vi "ACT_Loop.vi"() -> ()   [LabVIEW 2020, in "Wrist_ACT.lvlib"]
uses:
  Wrist_ACT.lvlib
  Cluster_CMD_ACT_Data.ctl
  Shared Code/TypeDefs/ENUM_Wrist_CMD_Mode Select.ctl
  Shared Code/TypeDefs/Cluster_Wrist_Config HW Values.ctl
  Shared Code/TypeDefs/Cluser_CAN Data.ctl
  Shared Code/TypeDefs/Cluster_Config Motor Output.ctl
  <vilib>/Rock Robotics/WPI/ThirdParty/Phoenix-LabVIEW/Motor Controller/Controls/CTRE_Phoenix_MotorControl_TalonFXInvertType.ctl
  <vilib>/Rock Robotics/WPI/ThirdParty/Phoenix-LabVIEW/Motor Controller/Controls/CTRE_Phoenix_MotorControl_NeutralMode.ctl
  Shared Code/TypeDefs/Cluster_FWD  REV Values.ctl
  Shared Code/TypeDefs/Cluster_PID Config.ctl
  Shared Code/TypeDefs/Cluster_PID Gains.ctl
  Shared Code/TypeDefs/Cluster_High-Low.ctl
  Shared Code/TypeDefs/Cluster_Motion Magic Parameters.ctl
  Shared Code/TypeDefs/Cluser_Limit Travel Config.ctl
  Shared Code/TypeDefs/Cluser_Hard Limits.ctl
  <vilib>/Rock Robotics/WPI/ThirdParty/Phoenix-LabVIEW/Motor Controller/Controls/CTRE_Phoenix_MotorControl_LimitSwitchNormal.ctl
  Shared Code/TypeDefs/Cluser_Config_Soft Limits.ctl
  Shared Code/TypeDefs/Cluser_Enable-Value I32.ctl
  Shared Code/TypeDefs/Cluster_Config_Cancoder Data.ctl
  Shared Code/TypeDefs/Cluser_Config_Current Limits.ctl
  Shared Code/TypeDefs/Cluster_Wrist HW Outputs.ctl
  Shared Code/TypeDefs/Cluster_FX Sensor Values.ctl
  Shared Code/TypeDefs/Cluster_FX CloseLoop Values.ctl
  Shared Code/TypeDefs/Cluster_FX Limit Switchs.ctl
  Shared Code/TypeDefs/Cluster_FX Current Values.ctl
  Shared Code/TypeDefs/Cluster_FX Integrated Sensor Values.ctl
  Shared Code/TypeDefs/Cluster_Wrist_SW Output Data.ctl
  Shared Code/TypeDefs/Cluster_Wrist_Config SW Values.ctl
  ENUM_ACT_State.ctl
  <vilib>/Rock Robotics/WPI/MotorControl/WPI_MotorControlDeviceRef.ctl
  <vilib>/Rock Robotics/WPI/MotorControl/WPI_MotorControlType.ctl
  <vilib>/Rock Robotics/SystemInterfaces/DIO/FPGA_DIOPWMChannel.ctl
  <vilib>/Rock Robotics/WPI/PWM/WPI_PWMDeadband.ctl
  <vilib>/Rock Robotics/SystemInterfaces/DIO/FPGA_DIOChannel.ctl
  <vilib>/Rock Robotics/WPI/ThirdParty/Phoenix-LabVIEW/Motor Controller/Controls/CTRE_Phoenix_MotorControl_ControlMode.ctl
  <vilib>/Rock Robotics/WPI/ThirdParty/Phoenix-LabVIEW/CANCoder/Controls/CTRE_Phoenix_CANcoder_DeviceRef.ctl
  ENUM_ACT_Action.ctl
  b65afb20-a57c-4a75-aa10-15f74f40a4cd.vi
  e7fa0f6b-fe57-4250-9995-b404d65a8362.vi
  4f1f8321-3dc8-4b28-8619-20673fc77ec2.vi
  6201c2b1-dcd8-4430-86f1-9b4ee56c7753.vi
  b5508d6c-c1cc-4273-80c5-2077d34e1483.vi
  36677ea0-a1a5-47a3-bc56-4475cb7c281e.vi
  5f725c2a-0ce1-4524-8967-e83b15fdce90.vi
  573e44c0-11f4-4bd9-ad56-904ec25dba75.vi
  e7494af9-f670-4352-9dfa-ae6ce50709ea.vi
  36677ea0-a1a5-47a3-bc56-4475cb7c281e.vi/f38ca901-adc1-4ad8-996e-31aeb746ae36.vi
  36677ea0-a1a5-47a3-bc56-4475cb7c281e.vi/958b2683-dd4b-41b7-8ed1-41c95f63cef0.vi
  5f725c2a-0ce1-4524-8967-e83b15fdce90.vi/f38ca901-adc1-4ad8-996e-31aeb746ae36.vi
  5f725c2a-0ce1-4524-8967-e83b15fdce90.vi/958b2683-dd4b-41b7-8ed1-41c95f63cef0.vi
  573e44c0-11f4-4bd9-ad56-904ec25dba75.vi/f38ca901-adc1-4ad8-996e-31aeb746ae36.vi
  573e44c0-11f4-4bd9-ad56-904ec25dba75.vi/958b2683-dd4b-41b7-8ed1-41c95f63cef0.vi
  e7494af9-f670-4352-9dfa-ae6ce50709ea.vi/f38ca901-adc1-4ad8-996e-31aeb746ae36.vi
  e7494af9-f670-4352-9dfa-ae6ce50709ea.vi/958b2683-dd4b-41b7-8ed1-41c95f63cef0.vi
  36677ea0-a1a5-47a3-bc56-4475cb7c281e.vi/f38ca901-adc1-4ad8-996e-31aeb746ae36.vi/1c6bd52c-bbca-4d4a-a290-93ea2703fded.vi
  36677ea0-a1a5-47a3-bc56-4475cb7c281e.vi/f38ca901-adc1-4ad8-996e-31aeb746ae36.vi/47c2b0d5-b5fa-444e-9535-611565d375db.vi
  5f725c2a-0ce1-4524-8967-e83b15fdce90.vi/f38ca901-adc1-4ad8-996e-31aeb746ae36.vi/1c6bd52c-bbca-4d4a-a290-93ea2703fded.vi
  5f725c2a-0ce1-4524-8967-e83b15fdce90.vi/f38ca901-adc1-4ad8-996e-31aeb746ae36.vi/47c2b0d5-b5fa-444e-9535-611565d375db.vi
  573e44c0-11f4-4bd9-ad56-904ec25dba75.vi/f38ca901-adc1-4ad8-996e-31aeb746ae36.vi/1c6bd52c-bbca-4d4a-a290-93ea2703fded.vi
  573e44c0-11f4-4bd9-ad56-904ec25dba75.vi/f38ca901-adc1-4ad8-996e-31aeb746ae36.vi/47c2b0d5-b5fa-444e-9535-611565d375db.vi
  e7494af9-f670-4352-9dfa-ae6ce50709ea.vi/f38ca901-adc1-4ad8-996e-31aeb746ae36.vi/1c6bd52c-bbca-4d4a-a290-93ea2703fded.vi
  e7494af9-f670-4352-9dfa-ae6ce50709ea.vi/f38ca901-adc1-4ad8-996e-31aeb746ae36.vi/47c2b0d5-b5fa-444e-9535-611565d375db.vi
  Utility/Global_STOP.vi
  Global_CMD_ACT_Data In.vi
  <vilib>/Utility/Data Type/Get Type Information.vi
  <vilib>/Utility/error.llb/Trim Whitespace.vi
  Shared Code/Utility/RWA/RWA/File/RWA_PC FIle Read String.vi
  Shared Code/Utility/RWA/RWA/Read Write Anything/RWA_File String.vi
  Shared Code/Utility/RWA/RWA/File/RWA_PC File Write String.vi
  <vilib>/Rock Robotics/WPI/ThirdParty/Phoenix-LabVIEW/CANCoder/Get/CTRE_Phoenix_CANcoder_GetSensorData.vi
  Global_ACT_Data Out.vi
  <vilib>/Comparison/Equal/Equal Functor/Equal Functor.lvclass
panel:
  in  "CMD Override":enum32{"None", "Velocity", "Position", "STOP"}(tab)
  in  "Velocity":dbl(slide) scale=-0.2..0.2
  in  "Target Counts":i32
  in  "Positon GO":bool
  out "Current Time":timestamp
  in  "SW Config":T1={"WristSW Ver"=0, "At Position Delay(S)"=0.2}
  out "SW Output":T2
  in  "Reset zero Offset on Limit Switch":bool
  out "Sensor Read time":dbl format="%.3g"
  out "HW Outputs":T3
  in  "Read Saved Config":bool
  in  "Update Config":bool
  in  "HW Config":T9 {"TravelLimits"."Soft"."REV"."Counts" format="%#.0f"; "TravelLimits"."Soft"."FWD"."Counts" format="%#.0f"; "Output"."Min"."REV" format="%.2f"; "Output"."Min"."FWD" format="%.2f"; "Output"."Max"."REV" format="%.2f"; "Output"."Max"."FWD" format="%.2f"; "CL"."Max I Accu"."Low" format="%#.8f"; "CL"."Max I Accu"."High" format="%#.8f"; "CL"."Gains"."F" format="%#.8f"; "CL"."Gains"."D" format="%#.8f"; "CL"."Gains"."I" format="%#.8f"; "CL"."Gains"."P" format="%#.8f"; "CL"."Error Allowed"."Low" format="%#.8f"; "CL"."Error Allowed"."High" format="%#.8f"; "CL"."I Zone"."Low" format="%#.8f"; "CL"."I Zone"."High" format="%#.8f"; "CL"."Max Out"."REV" format="%.2f"; "CL"."Max Out"."FWD" format="%.2f"}
  out "CMD":T26
  out "Cycle Time (S)":dbl format="%.3g"
  # "STOP"
  # "Tune Output\nto 1023 Max"
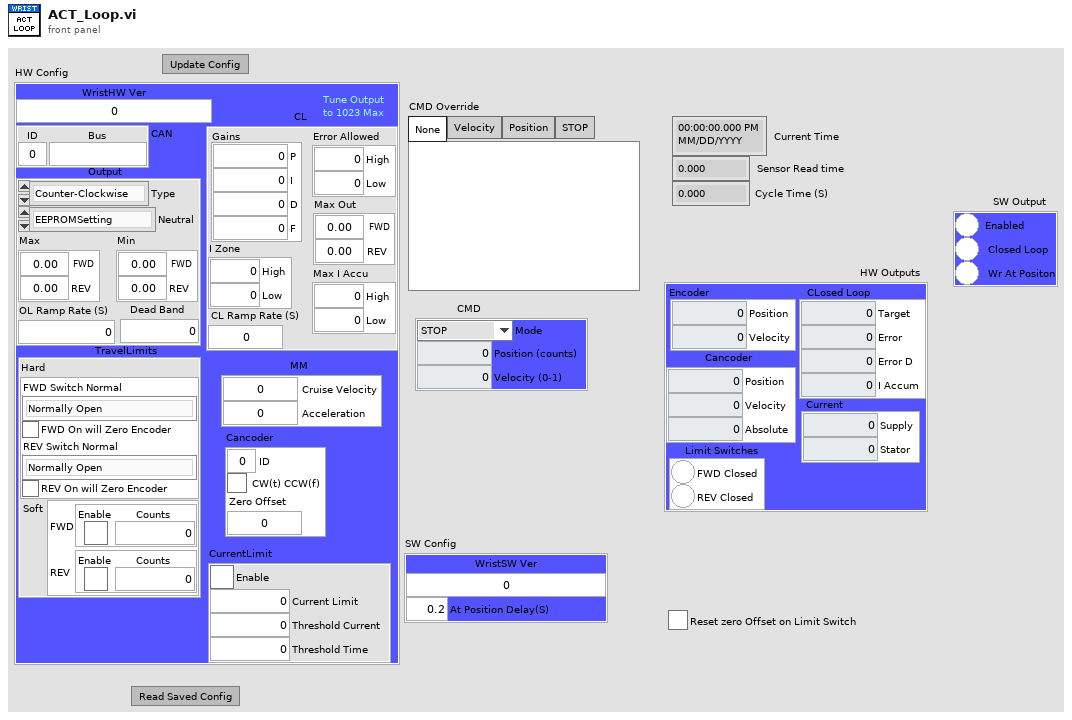
[diagram p1: front panel]
types:
  T1 = typedef "Cluster_Wrist_Config SW Values.ctl" = cluster{"WristSW Ver":u64, "At Position Delay(S)":dbl}
  T2 = typedef "Cluster_Wrist_SW Output Data.ctl" = cluster{"Enabled":bool, "Closed Loop":bool, "Wr At Positon":bool}
  T3 = typedef "Cluster_Wrist HW Outputs.ctl" = cluster{"Encoder":T4, "CLosed Loop":T5, "Limit Switches":T6, "Current":T7, "Cancoder":T8}
  T4 = typedef "Cluster_FX Sensor Values.ctl" = cluster{"Position":i32, "Velocity":i32}
  T5 = typedef "Cluster_FX CloseLoop Values.ctl" = cluster{"Target":dbl, "Error":i32, "Error D":dbl, "I Accum":dbl}
  T6 = typedef "Cluster_FX Limit Switchs.ctl" = cluster{"FWD Closed":bool, "REV Closed":bool}
  T7 = typedef "Cluster_FX Current Values.ctl" = cluster{"Supply":dbl, "Stator":dbl}
  T8 = typedef "Cluster_FX Integrated Sensor Values.ctl" = cluster{"Position":dbl, "Velocity":dbl, "Absolute":dbl}
  T9 = typedef "Cluster_Wrist_Config HW Values.ctl" = cluster{"WristHW Ver":u64, "CAN":T10, "Output":T11, "CL":T15, "MM":T18, "TravelLimits":T19, "Cancoder":T24, "CurrentLimit":T25}
  T10 = typedef "Cluser_CAN Data.ctl" = cluster{"ID":u8, "Bus":string}
  T11 = typedef "Cluster_Config Motor Output.ctl" = cluster{"Type":T12, "Neutral":T13, "Max":T14, "Min":T14, "OL Ramp Rate (S)":dbl, "Dead Band":dbl}
  T12 = typedef "CTRE_Phoenix_MotorControl_TalonFXInvertType.ctl" = enum16{"Counter-Clockwise", "Clockwise"}
  T13 = typedef "CTRE_Phoenix_MotorControl_NeutralMode.ctl" = enum8{"EEPROMSetting", "Override to Coast", "Override to Brake"}
  T14 = typedef "Cluster_FWD  REV Values.ctl" = cluster{"FWD":dbl, "REV":dbl}
  T15 = typedef "Cluster_PID Config.ctl" = cluster{"Gains":T16, "Error Allowed":T17, "I Zone":T17, "Max Out":T14, "Max I Accu":T17, "CL Ramp Rate (S)":dbl}
  T16 = typedef "Cluster_PID Gains.ctl" = cluster{"P":dbl, "I":dbl, "D":dbl, "F":dbl}
  T17 = typedef "Cluster_High-Low.ctl" = cluster{"High":dbl, "Low":dbl}
  T18 = typedef "Cluster_Motion Magic Parameters.ctl" = cluster{"Cruise Velocity":i32, "Acceleration":i32}
  T19 = typedef "Cluser_Limit Travel Config.ctl" = cluster{"Hard":T20, "Soft":T22}
  T20 = typedef "Cluser_Hard Limits.ctl" = cluster{"FWD Switch Normal":T21, "FWD On will Zero Encoder ":bool, "REV Switch Normal":T21, "REV On will Zero Encoder ":bool}
  T21 = typedef "CTRE_Phoenix_MotorControl_LimitSwitchNormal.ctl" = enum16{"Normally Open", "Normally Closed", "Disabled"}
  T22 = typedef "Cluser_Config_Soft Limits.ctl" = cluster{"FWD":T23, "REV":T23}
  T23 = typedef "Cluser_Enable-Value I32.ctl" = cluster{"Enable":bool, "Counts":i32}
  T24 = typedef "Cluster_Config_Cancoder Data.ctl" = cluster{"ID":u8, "CW(t) CCW(f)":bool, "Zero Offset":dbl}
  T25 = typedef "Cluser_Config_Current Limits.ctl" = cluster{"Enable":bool, "Current Limit":dbl, "Threshold Current":dbl, "Threshold Time":dbl}
  T26 = typedef "Wrist_ACT.lvlib/Cluster_CMD_ACT_Data.ctl" = cluster{"Mode":T27, "Position (counts)":i32, "Velocity (0-1)":dbl}
  T27 = typedef "ENUM_Wrist_CMD_Mode Select.ctl" = enum16{"STOP", "Position", "Speed"}
  T28 = typedef "CTRE_Phoenix_CANcoder_DeviceRef.ctl" = cluster{"DeviceStatus":errorcluster, "Device Number":u8, "Handle":u64, "UsageFrame":u32, "Library Path":path}
  T29 = typedef "CTRE_Phoenix_MotorControl_ControlMode.ctl" = u16
  T30 = typedef "WPI_MotorControlDeviceRef.ctl" = cluster{"DeviceStatus":errorcluster, "Type":T31, "PWM":cluster{"PWM Channel":T32, "DeadBand":T33}, "CAN":cluster{"Device Number":u8, "SetOutput VI Ref":variant, "GetOutput VI Ref":variant, "Enable VI Ref":variant, "Disable VI Ref":variant, "Data":variant}, "Invert":bool, "DIO PWM":cluster{"PWM \"Enable\" Channel":T32, "DIOChannel":T34, "PWM Rate":dbl}}
  T31 = typedef "WPI_MotorControlType.ctl" = enum16{"PWM", "CAN", "DIO PWM"}
  T32 = typedef "FPGA_DIOPWMChannel.ctl" = enum8{"PWM 0", "PWM 1", "PWM 2", "PWM 3", "PWM 4", "PWM 5", "PWM 6", "PWM 7", "PWM 8", "PWM 9", "PWM MXP 0", "PWM MXP 1", "PWM MXP 2", "PWM MXP 3", "PWM MXP 4", "PWM MXP 5", "PWM MXP 6", "PWM MXP 7", "PWM MXP 8", "PWM MXP 9", "Invalid"}
  T33 = typedef "WPI_PWMDeadband.ctl" = cluster{"Name":string, "maxPositivePwm":i32, "minPositivePwm":i32, "centerPwm":i32, "maxNegativePwm":i32, "minNegativePwm":i32, "angularRange":u16}
  T34 = typedef "FPGA_DIOChannel.ctl" = enum8{"DIO 0", "DIO 1", "DIO 2", "DIO 3", "DIO 4", "DIO 5", "DIO 6", "DIO 7", "DIO 8", "DIO 9", "DIO MXP 0", "DIO MXP 1", "DIO MXP 2", "DIO MXP 3", "DIO MXP 4", "DIO MXP 5", "DIO MXP 6", "DIO MXP 7", "DIO MXP 8", "DIO MXP 9", "DIO MXP 10", "DIO MXP 11", "DIO MXP 12", "DIO MXP 13", "DIO MXP 14", "DIO MXP 15", "SPI Port CS1", "SPI Port CS2", "SPI Port CS3", "SPI Port MISO", "SPI Port MOSI", "Invalid"}
  T35 = typedef "Wrist_ACT.lvlib/ENUM_ACT_State.ctl" = enum16{"Startup", "Configuring", "Stopping", "Moving Position", "Moving Velocity", "Shutdown"}
  T36 = cluster{"Falcon Ref":T30, "State":T35, "Previous State":T35, "Current Time":timestamp, "Previous Time":timestamp, "Start Time":timestamp, "Target Time (ms)":u32, "Cycle Time(S)":dbl, "ACT Input":T26, "ACT Output DBL":dbl, "Team Files Folder":path, "HW Config":T9, "Update Display":bool, "Max # Of Config Tries":i32, "CAN Timeout":u32, "FX Mode":T29, "FX Set Value":dbl, "HW Outputs":T3, "CANcoder Ref":T28, "SW Outputs":T2, "SW Config":T1}
  T37 = typedef "Wrist_ACT.lvlib/ENUM_ACT_Action.ctl" = enum16{"No Action", "Reset Time", "Reset All", "Config HW File Read", "Config HW File Save", "Config SW File Read", "Config SW File Save", "Config From FP", "Config HW Get", "Config HW Set", "Open HW Only", "Control FX Stop", "Control FX Positon", "Control FX Speed", "Config Cancoder Get Offset Value"}
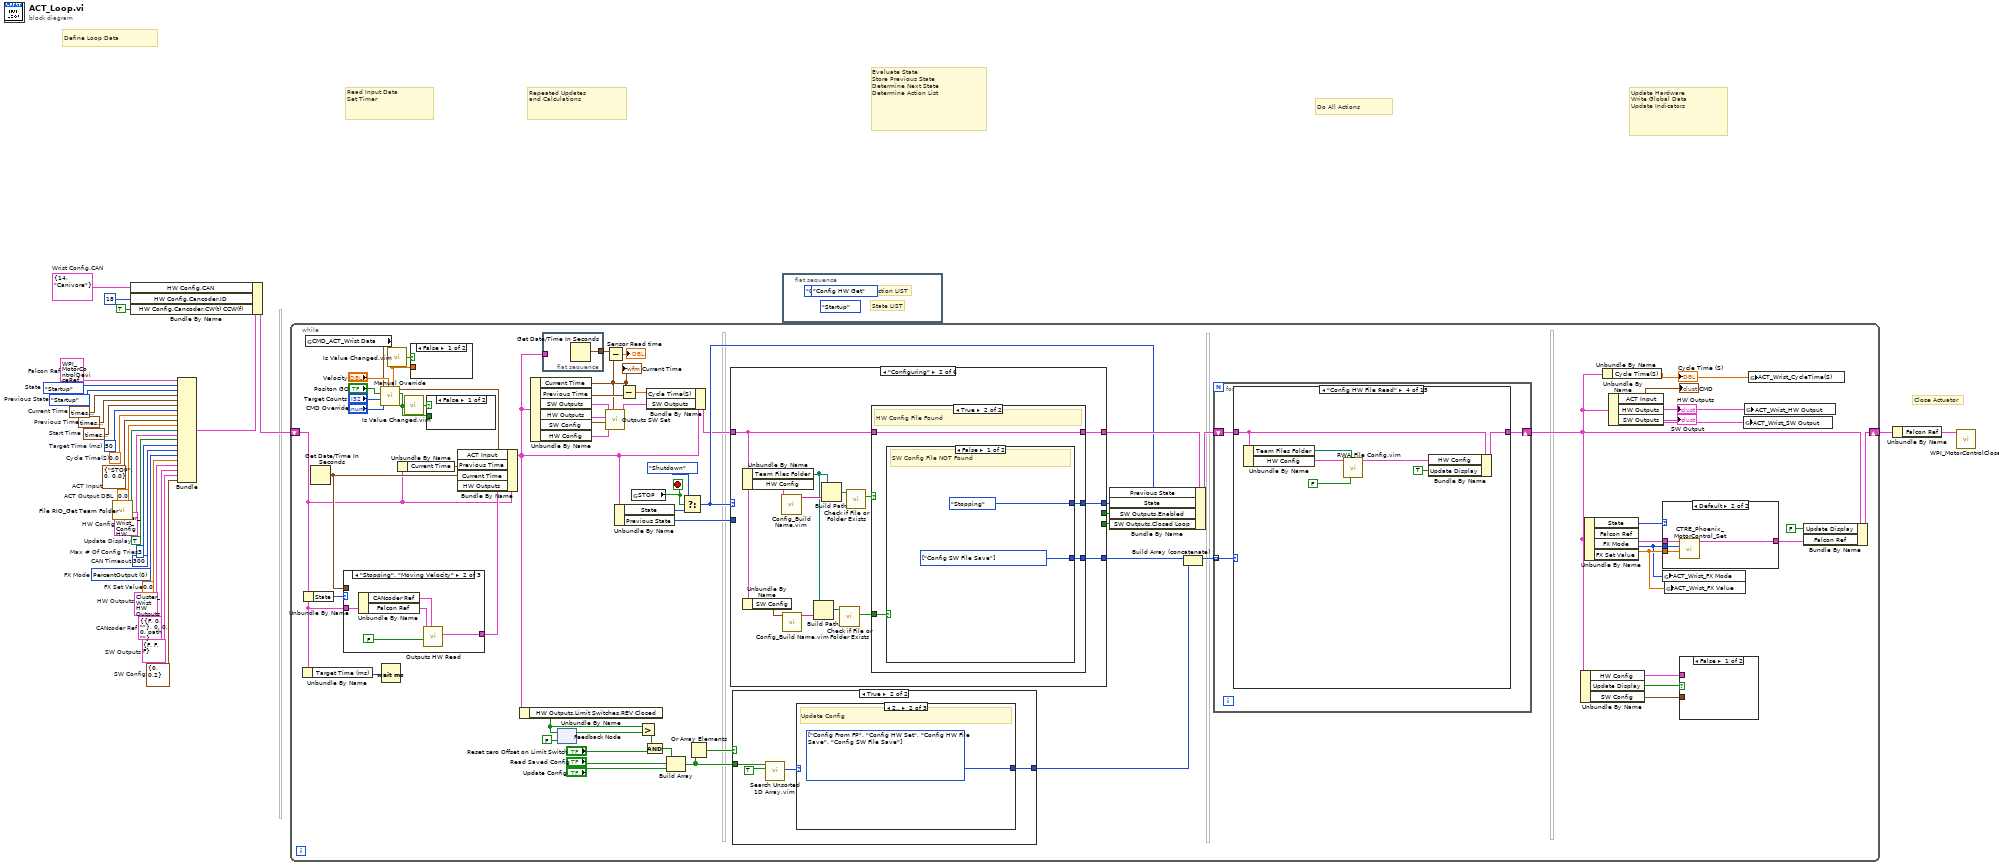
[diagram p0: block diagram]
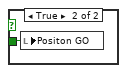
[diagram p2: hidden frame]
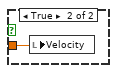
[diagram p3: hidden frame]
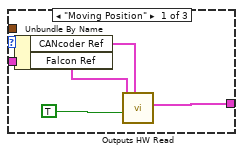
[diagram p4: hidden frame]
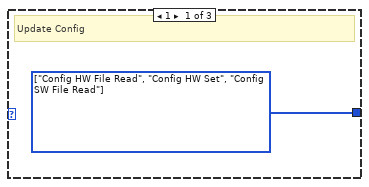
[diagram p7: hidden frame]
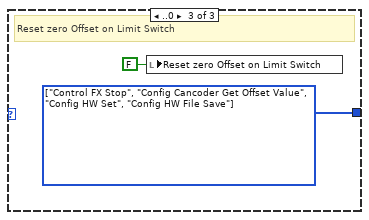
[diagram p8: hidden frame]
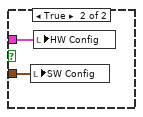
[diagram p10: hidden frame]
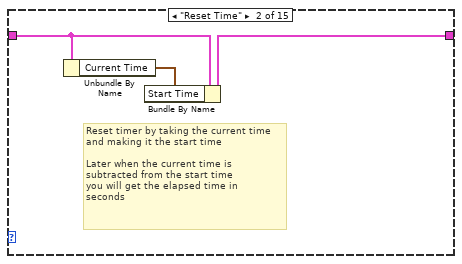
[diagram p12: hidden frame]
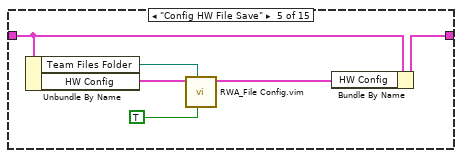
[diagram p14: hidden frame]
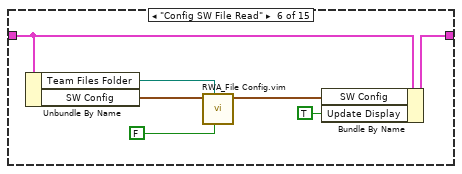
[diagram p15: hidden frame]
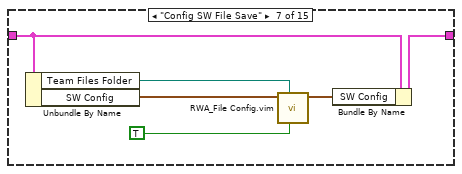
[diagram p16: hidden frame]
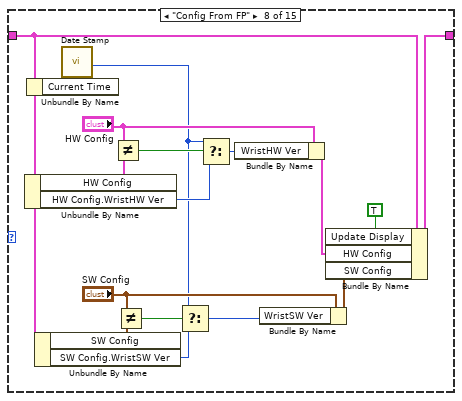
[diagram p17: hidden frame]
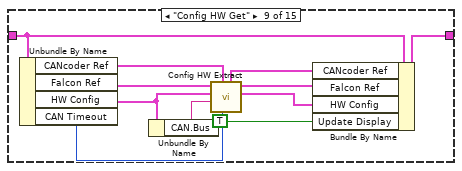
[diagram p18: hidden frame]
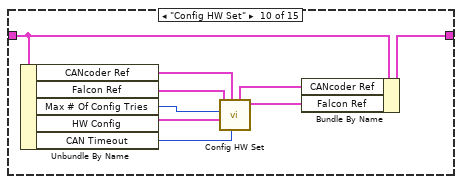
[diagram p19: hidden frame]
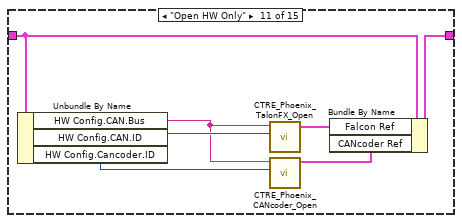
[diagram p20: hidden frame]
diagram:
  w1 = T1 {"WristSW Ver"=0, "At Position Delay(S)"=0.2}  # SW Config
  w2 = T2 {"Enabled"=FALSE, "Closed Loop"=FALSE, "Wr At Positon"=FALSE}  # SW Outputs
  w5 = T28 {"DeviceStatus"={"status"=FALSE, "code"=0, "source"=""}, "Device Number"=0, "Handle"=0, "UsageFrame"=0, "Library Path"=path ""}  # CANcoder Ref
  w6 = T3 {"Encoder"={"Position"=0, "Velocity"=0}, "CLosed Loop"={"Target"=0.0, "Error"=0, "Error D"=0.0, "I Accum"=0.0}, "Limit Switches"={"FWD Closed"=FALSE, "REV Closed"=FALSE}, "Current"={"Supply"=0.0, "Stator"=0.0}, "Cancoder"={"Position"=0.0, "Velocity"=0.0, "Absolute"=0.0}}  # HW Outputs
  w8 = 0.0  # FX Set Value
  w9 = T29 0 items=["PercentOutput"=0, "Position"=1, "Velocity"=2, "Current"=3, "Follower"=5, "MotionProfile"=6, "MotionMagic"=7, "MotionProfileArc"=10, "Disabled"=15]  # FX Mode
  w10 = u32 300  # CAN Timeout
  w11 = 3  # Max # Of Config Tries
  w12 = TRUE  # Update Display
  w13 = T10 {"ID"=14, "Bus"="Canivore"}  # Wrist Config.CAN
  w14 = T9 {"WristHW Ver"=0, "CAN"={"ID"=0, "Bus"=""}, "Output"={"Type"=enum."Counter-Clockwise", "Neutral"=enum."EEPROMSetting", "Max"={"FWD"=0.0, "REV"=0.0}, "Min"={"FWD"=0.0, "REV"=0.0}, "OL Ramp Rate (S)"=0.0, "Dead Band"=0.0}, "CL"={"Gains"={"P"=0.0, "I"=0.0, "D"=0.0, "F"=0.0}, "Error Allowed"={"High"=0.0, "Low"=0.0}, "I Zone"={"High"=0.0, "Low"=0.0}, "Max Out"={"FWD"=0.0, "REV"=0.0}, "Max I Accu"={"High"=0.0, "Low"=0.0}, "CL Ramp Rate (S)"=0.0}, "MM"={"Cruise Velocity"=0, "Acceleration"=0}, "TravelLimits"={"Hard"={"FWD Switch Normal"=enum."Normally Open", "FWD On will Zero Encoder "=FALSE, "REV Switch Normal"=enum."Normally Open", "REV On will Zero Encoder "=FALSE}, "Soft"={"FWD"={"Enable"=FALSE, "Counts"=0}, "REV"={"Enable"=FALSE, "Counts"=0}}}, "Cancoder"={"ID"=0, "CW(t) CCW(f)"=FALSE, "Zero Offset"=0.0}, "CurrentLimit"={"Enable"=FALSE, "Current Limit"=0.0, "Threshold Current"=0.0, "Threshold Time"=0.0}}  # HW Config
  w16 = T30 {"DeviceStatus"={"status"=FALSE, "code"=0, "source"=""}, "Type"=enum."PWM", "PWM"={"PWM Channel"=enum."PWM 1", "DeadBand"={"Name"="", "maxPositivePwm"=0, "minPositivePwm"=0, "centerPwm"=0, "maxNegativePwm"=0, "minNegativePwm"=0, "angularRange"=0}}, "CAN"={"Device Number"=0, "SetOutput VI Ref"=variant(enum8{"Percent VBus", "Current", "Speed", "Position", "Voltage"} enum."Percent VBus"), "GetOutput VI Ref"=variant(refnum<k1> refnum), "Enable VI Ref"=variant(dbl 12.0), "Disable VI Ref"=variant(enum8{"Percent VBus", "Speed", "Position", "Slave", "Unchanged / Invalid", "Voltage Compensation", "Current", "Motion Profile"} enum."Percent VBus"), "Data"=variant}, "Invert"=FALSE, "DIO PWM"={"PWM \"Enable\" Channel"=enum."Invalid", "DIOChannel"=enum."Invalid", "PWM Rate"=0.0}}  # Falcon Ref
  w20 = 0.0  # Cycle Time(S)
  w21 = ENUM_ACT_State."Startup"  # Previous State
  w22 = timestamp(0 s since 1904-01-01)  # Previous Time
  w23 = u32 50  # Target Time (ms)
  w24 = 0.0  # ACT Output DBL
  w25 = T26 {"Mode"=enum."STOP", "Position (counts)"=0, "Velocity (0-1)"=0.0}  # ACT Input
  w26 = timestamp(0 s since 1904-01-01)  # Start Time
  w27 = timestamp(0 s since 1904-01-01)  # Current Time
  w28 = ENUM_ACT_State."Startup"  # State
  # "Close Actuator"
  # "Define Loop Data"
  # "Repeated Updates\nand Calculations"
  # "Read Input Data\nSet Timer"
  # "Evaluate State\nStore Previous State\nDetermine Next State\nDetermine Action List"
  # "Do All Actions"
  # "Update Hardware\nWrite Global Data\nUpdate Indicators"
  n1 = call "File RIO_Get Team Folder.vi"() -> ("Team Files Folder"=w15:path)  [unwired: 10 in, 1 out]
  n2 = Bundle("Falcon Ref"=w16, "State"=w28, "Previous State"=w21, "Current Time"=w27, "Previous Time"=w22, "Start Time"=w26, "Target Time (ms)"=w23, "Cycle Time(S)"=w20, "ACT Input"=w25, "ACT Output DBL"=w24, "Team Files Folder"=w15, "HW Config"=w14, "Update Display"=w12, "Max # Of Config Tries"=w11, "CAN Timeout"=w10, "FX Mode"=w9, "FX Set Value"=w8, "HW Outputs"=w6, "CANcoder Ref"=w5, "SW Outputs"=w2, "SW Config"=w1) -> (w18:T36)  [unwired: 1 in]
  n3 = Bundle By Name(cluster=w18, "HW Config.CAN"=w13, "HW Config.Cancoder.ID"=u8 18 ("Wrist Config.Cancoder.ID"), "HW Config.Cancoder.CW(t) CCW(f)"=TRUE ("Wrist Config.Cancoder.CW(t) CCW(f)")) -> (w17:T36)
  n4 = while {
    shift-right: [w77] -> w19
    shift-left: w17 -> [w39]
    stop <- w91 stop-if-true
    n5 = Unbundle By Name(w39) -> ("Target Time (ms)"=w88:u32)
    n6 = Unbundle By Name(w39) -> ("State"=w67:T35)
    n7 = global read "Global_CMD_ACT_Data In.vi" "CMD_ACT_Wrist Data"() -> (w29:T26)
    n8 = Get Date/Time In Seconds() -> (seconds since 1Jan1904=w63:timestamp)
    n9 = case shown="\"Stopping\", \"Moving Velocity\"" w67 {
      tunnel: w39 -> [w102 w107 _]
      tunnel: w63 -> [_ _ _]
      tunnel: [w99 w104 _] -> w40
      frame "Moving Position" {
        n10 = Unbundle By Name(w102) -> ("CANcoder Ref"=w98:T28, "Falcon Ref"=w101:T30)
        n11 = call "Outputs HW Read.vi"("CTRE_CANcoder_DeviceRef"=w98, "Read Closed Loop"=TRUE, "Ref"=w101) -> ("Sensor Values Out"=w99:T3)  [unwired: 5 in, 3 out]
      }
      frame "Stopping", "Moving Velocity" {
        n12 = Unbundle By Name(w107) -> ("CANcoder Ref"=w103:T28, "Falcon Ref"=w106:T30)
        n13 = call "Outputs HW Read.vi"("CTRE_CANcoder_DeviceRef"=w103, "Read Closed Loop"=FALSE, "Ref"=w106) -> ("Sensor Values Out"=w104:T3)  [unwired: 5 in, 3 out]
      }
      frame "Startup", "Configuring", "Shutdown" {
      }
    }
    n14 = call "Manual Override.vi"("Velocity"="Velocity", "Override"="CMD Override", "Counts"="Target Counts", "Position GO"="Positon GO", "Auto CMD"=w29) -> ("Position GO Out"=w36:bool, "OverRide Command Out"=w30:T26, "Velocity Out"=w34:dbl)  [unwired: 4 in]
    n15 = Wait (ms)(milliseconds to wait=w88) -> ()  [unwired: 1 out]
    n16 = call "Is Value Changed.vim"("value"=w34) -> ("changed or first call?"=w35:bool)
    n17 = Unbundle By Name(w39) -> ("Current Time"=w87:timestamp)
    n18 = call "Is Value Changed.vim"("value"=w36) -> ("changed or first call?"=w37:bool)
    n19 = case shown="False" w35 {
      tunnel: w34 -> [_ w96]
      frame False {
      }
      frame True {
        n20 = local write "Velocity"(w96) -> ()
      }
    }
    n21 = case shown="False" w37 {
      tunnel: w36 -> [_ w95]
      frame False {
      }
      frame True {
        n22 = local write "Positon GO"(w95) -> ()
      }
    }
    n23 = Bundle By Name(cluster=w39, "ACT Input"=w30, "Previous Time"=w87, "Current Time"=w63, "HW Outputs"=w40) -> (w41:T36)
    n24 = Unbundle By Name(w41) -> ("HW Outputs.Limit Switches.REV Closed"=w56:bool)
    n25 = Unbundle By Name(w41) -> ("Current Time"=w45:timestamp, "Previous Time"=w84:timestamp, "SW Outputs"=w48:T2, "HW Outputs"=w46:T3, "SW Config"=w44:T1, "HW Config"=w43:T9)
    "Current Time" <- w45
    n26 = flat-sequence {
      tunnel: [w97] -> w65
      tunnel: w41 -> [_]
      frame #0 {
        n27 = Get Date/Time In Seconds() -> (seconds since 1Jan1904=w97:timestamp)
      }
    }
    n28 = feedback #1(FALSE ("REV Closed")) -> (w57:bool)
    n29 = feedback-in #1(w56) -> ()
    n30 = call "Outputs SW Set.vi"("Current Time"=w45, "Wrist Config"=w43, "WristSW Config"=w44, "Sensor Values"=w46, "SW Output"=w48) -> ("SW Output Out"=w47:T2)  [unwired: 6 in]
    n31 = Subtract(x=w65, y=w45) -> (x-y=→"Sensor Read time":dbl)
    n32 = Unbundle By Name(w41) -> ("State"=w89:T35, "Previous State"=w86:T35)
    n33 = Subtract(x=w45, y=w84) -> (x-y=w82:dbl)
    n34 = global read "Global_STOP.vi" "STOP"() -> (w91:bool)
    n35 = Greater?(x=w56, y=w57) -> (0:w54:bool)
    n36 = And(x=w54, y="Reset zero Offset on Limit Switch") -> (x .and. y?=w53:bool)
    n37 = Bundle By Name(cluster=w41, "Cycle Time(S)"=w82, "SW Outputs"=w47) -> (w83:T36)
    n38 = Build Array(w53, "Read Saved Config", "Update Config") -> (w59:bool[])
    n39 = Select(t=ENUM_ACT_State."Shutdown" ("State"), s=w91, f=w89) -> (s? t:f=w85:T35)
    n40 = Or Array Elements(Boolean array=w59) -> (logical OR=w60:bool)
    n41 = case shown="\"Configuring\"" w85 {
      selector: w85 -> [_ _ _ w265 w282 _]
      tunnel: w83 -> [w221 w227 w251 w266 w283 w298]
      tunnel: [w221 w230 w250 w267 w284 w298] -> w93
      tunnel: [ENUM_ACT_State."Configuring" ("State") w229 w249 w269 w286 ENUM_ACT_State."Shutdown" ("State")] -> w92
      tunnel: [w220 w228 w247 w264 w280 w296] -> w81
      tunnel: w86 -> [_ _ _ _ _ _]
      tunnel: [_ _ TRUE w262 TRUE _] -> w50
      tunnel: [_ _ _ w262 _ _] -> w49
      frame "Startup" {
        w220 = T37[] [enum."Reset Time"] items=["No Action", "Reset Time", "Reset All", "Config HW File Read", "Config HW File Save", "Config SW File Read", "Config SW File Save", "Config From FP", "Config HW Get", "Config HW Set", "Open HW Only", "Control FX Stop", "Control FX Positon", "Control FX Speed", "Config Cancoder Get Offset Value"] ("Actions")
      }
      frame "Configuring" {
        n42 = Unbundle By Name(w227) -> ("Team Files Folder"=w224:path, "HW Config"=w232:T9)
        n43 = Unbundle By Name(w227) -> ("SW Config"=w225:T1)
        n44 = call "Config_Build Name.vim"("Config First Name"=w232) -> ("Cfg file"=w234:string)  [unwired: 9 in, 1 out]
        n45 = call "Config_Build Name.vim"("Config First Name"=w225) -> ("Cfg file"=w226:string)  [unwired: 9 in, 1 out]
        n46 = Build Path(base path=w224, name or relative path=w226) -> (appended path=w223:path)
        n47 = Build Path(base path=w224, name or relative path=w234) -> (appended path=w233:path)
        n48 = call <vilib>:"Check if File or Folder Exists.vi"("path"=w223) -> ("file or folder exists?"=w222:bool)  [unwired: 8 in, 2 out]
        n49 = call <vilib>:"Check if File or Folder Exists.vi"("path"=w233) -> ("file or folder exists?"=w231:bool)  [unwired: 8 in, 2 out]
        n50 = case shown="True" w231 {
          tunnel: w227 -> [w237 w241]
          tunnel: [w237 w241] -> w230
          tunnel: [ENUM_ACT_State."Configuring" ("State") w240] -> w229
          tunnel: [w235 w239] -> w228
          tunnel: w222 -> [_ w238]
          frame False {
            w235 = T37[] [enum."Open HW Only", enum."Config HW Get", enum."Config HW File Save"] items=["No Action", "Reset Time", "Reset All", "Config HW File Read", "Config HW File Save", "Config SW File Read", "Config SW File Save", "Config From FP", "Config HW Get", "Config HW Set", "Open HW Only", "Control FX Stop", "Control FX Positon", "Control FX Speed", "Config Cancoder Get Offset Value"] ("Actions")
            # "HW Config File Not Found"
          }
          frame True {
            # "HW Config File Found"
            n51 = case shown="False" w238 {
              tunnel: [ENUM_ACT_State."Stopping" ("State") ENUM_ACT_State."Stopping" ("State")] -> w240
              tunnel: [w242 w244] -> w239
              frame False {
                w242 = T37[] [enum."Config SW File Save"] items=["No Action", "Reset Time", "Reset All", "Config HW File Read", "Config HW File Save", "Config SW File Read", "Config SW File Save", "Config From FP", "Config HW Get", "Config HW Set", "Open HW Only", "Control FX Stop", "Control FX Positon", "Control FX Speed", "Config Cancoder Get Offset Value"] ("Actions")
                # "SW Config File NOT Found"
              }
              frame True {
                w244 = T37[] [enum."Config HW File Read", enum."Config HW Set", enum."Config SW File Read", enum."Reset All", enum."Control FX Stop"] items=["No Action", "Reset Time", "Reset All", "Config HW File Read", "Config HW File Save", "Config SW File Read", "Config SW File Save", "Config From FP", "Config HW Get", "Config HW Set", "Open HW Only", "Control FX Stop", "Control FX Positon", "Control FX Speed", "Config Cancoder Get Offset Value"] ("Actions")
                # "SW Config File Found"
              }
            }
          }
        }
      }
      frame "Stopping" {
        w248 = T37[] [enum."Control FX Stop"] items=["No Action", "Reset Time", "Reset All", "Config HW File Read", "Config HW File Save", "Config SW File Read", "Config SW File Save", "Config From FP", "Config HW Get", "Config HW Set", "Open HW Only", "Control FX Stop", "Control FX Positon", "Control FX Speed", "Config Cancoder Get Offset Value"] ("Actions")
        n52 = Unbundle By Name(w251) -> ("ACT Input.Mode"=w252:T27)
        n53 = case shown="\"STOP\"" w252 {
          tunnel: w251 -> [w255 w258 w261]
          tunnel: [w255 w258 w261] -> w250
          tunnel: [ENUM_ACT_State."Stopping" ("State") ENUM_ACT_State."Moving Position" ("State") ENUM_ACT_State."Moving Velocity" ("State")] -> w249
          tunnel: [w253 w256 w259] -> w247
          tunnel: w248 -> [w253 w256 w259]
          frame "STOP" {
          }
          frame "Position" {
          }
          frame "Speed" {
          }
        }
      }
      frame "Moving Position" {
        w262 = TRUE
        w263 = T37[] [enum."Control FX Stop"] items=["No Action", "Reset Time", "Reset All", "Config HW File Read", "Config HW File Save", "Config SW File Read", "Config SW File Save", "Config From FP", "Config HW Get", "Config HW Set", "Open HW Only", "Control FX Stop", "Control FX Positon", "Control FX Speed", "Config Cancoder Get Offset Value"] ("Actions")
        n54 = Unbundle By Name(w266) -> ("ACT Input.Mode"=w268:T27)
        n55 = case shown="\"Speed\"" w268 {
          tunnel: [ENUM_ACT_State."Stopping" ("State") ENUM_ACT_State."Moving Velocity" ("State") w277] -> w269
          tunnel: w266 -> [w272 w275 w278]
          tunnel: [w272 w275 w278] -> w267
          tunnel: w265 -> [_ _ w277]
          tunnel: [w270 w273 w276] -> w264
          tunnel: w263 -> [w270 w273 _]
          frame "STOP" {
          }
          frame "Speed" {
          }
          frame "Position" {
            w276 = T37[] [enum."Control FX Positon"] items=["No Action", "Reset Time", "Reset All", "Config HW File Read", "Config HW File Save", "Config SW File Read", "Config SW File Save", "Config From FP", "Config HW Get", "Config HW Set", "Open HW Only", "Control FX Stop", "Control FX Positon", "Control FX Speed", "Config Cancoder Get Offset Value"] ("Actions")
          }
        }
      }
      frame "Moving Velocity" {
        w281 = T37[] [enum."Control FX Stop"] items=["No Action", "Reset Time", "Reset All", "Config HW File Read", "Config HW File Save", "Config SW File Read", "Config SW File Save", "Config From FP", "Config HW Get", "Config HW Set", "Open HW Only", "Control FX Stop", "Control FX Positon", "Control FX Speed", "Config Cancoder Get Offset Value"] ("Actions")
        n56 = Unbundle By Name(w283) -> ("ACT Input.Mode"=w285:T27)
        n57 = case shown="\"STOP\"" w285 {
          tunnel: [ENUM_ACT_State."Stopping" ("State") w290 ENUM_ACT_State."Moving Position" ("State")] -> w286
          tunnel: w283 -> [w289 w292 w295]
          tunnel: [w289 w292 w295] -> w284
          tunnel: w282 -> [_ w290 _]
          tunnel: [w287 w291 w293] -> w280
          tunnel: w281 -> [w287 _ w293]
          frame "STOP" {
          }
          frame "Speed" {
            w291 = T37[] [enum."Control FX Speed"] items=["No Action", "Reset Time", "Reset All", "Config HW File Read", "Config HW File Save", "Config SW File Read", "Config SW File Save", "Config From FP", "Config HW Get", "Config HW Set", "Open HW Only", "Control FX Stop", "Control FX Positon", "Control FX Speed", "Config Cancoder Get Offset Value"] ("Actions")
          }
          frame "Position" {
          }
        }
      }
      frame "Shutdown" {
        w296 = T37[] [enum."Reset All"] items=["No Action", "Reset Time", "Reset All", "Config HW File Read", "Config HW File Save", "Config SW File Read", "Config SW File Save", "Config From FP", "Config HW Get", "Config HW Set", "Open HW Only", "Control FX Stop", "Control FX Positon", "Control FX Speed", "Config Cancoder Get Offset Value"] ("Actions")
      }
    }
    n58 = case shown="True" w60 {
      tunnel: w59 -> [_ w110]
      tunnel: [_ w108] -> w58
      frame False {
      }
      frame True {
        n59 = call "Search Unsorted 1D Array.vim"("element"=TRUE, "unsorted 1D array"=w110) -> ("index of element"=w109:i32)  [unwired: 9 in]
        n60 = case shown="2.." w109 {
          tunnel: [w112 w113 w115] -> w108
          frame 1 {
            w112 = T37[] [enum."Config HW File Read", enum."Config HW Set", enum."Config SW File Read"] items=["No Action", "Reset Time", "Reset All", "Config HW File Read", "Config HW File Save", "Config SW File Read", "Config SW File Save", "Config From FP", "Config HW Get", "Config HW Set", "Open HW Only", "Control FX Stop", "Control FX Positon", "Control FX Speed", "Config Cancoder Get Offset Value"] ("Actions")
            # "Update Config"
          }
          frame 2.. {
            w113 = T37[] [enum."Config From FP", enum."Config HW Set", enum."Config HW File Save", enum."Config SW File Save"] items=["No Action", "Reset Time", "Reset All", "Config HW File Read", "Config HW File Save", "Config SW File Read", "Config SW File Save", "Config From FP", "Config HW Get", "Config HW Set", "Open HW Only", "Control FX Stop", "Control FX Positon", "Control FX Speed", "Config Cancoder Get Offset Value"] ("Actions")
            # "Update Config"
          }
          frame ..0 {
            w115 = T37[] [enum."Control FX Stop", enum."Config Cancoder Get Offset Value", enum."Config HW Set", enum."Config HW File Save"] items=["No Action", "Reset Time", "Reset All", "Config HW File Read", "Config HW File Save", "Config SW File Read", "Config SW File Save", "Config From FP", "Config HW Get", "Config HW Set", "Open HW Only", "Control FX Stop", "Control FX Positon", "Control FX Speed", "Config Cancoder Get Offset Value"] ("Actions")
            # "Reset zero Offset on Limit Switch"
            n61 = local write "Reset zero Offset on Limit Switch"(FALSE ("Reset zero Offset on Limit Switch")) -> ()
          }
        }
      }
    }
    n62 = Bundle By Name(cluster=w93, "Previous State"=w85, "State"=w92, "SW Outputs.Enabled"=w50, "SW Outputs.Closed Loop"=w49) -> (w94:T36)
    n63 = Build Array (concatenate)(w81, w58) -> (w75:T37[])
    n64 = for {
      tunnel: w75 -> [w125] mode=indexing
      shift-right: [w124] -> w74
      shift-left: w94 -> [w123]
      n65 = case shown="\"Config HW File Read\"" w125 {
        tunnel: w123 -> [w126 w129 w130 w136 w142 w149 w155 w163 w180 w191 w197 w203 w206 w211 w216]
        tunnel: [w126 w128 w130 w137 w143 w150 w156 w173 w181 w192 w198 w204 w208 w213 w217] -> w124
        frame "No Action" {
        }
        frame "Reset Time" {
          # "Reset timer by taking the current time\nand making it the start time\n\nLater when the current time is \nsubtracted from the start time\nyou will get the elapsed time in \nseconds"
          n66 = Unbundle By Name(w129) -> ("Current Time"=w127:timestamp)
          n67 = Bundle By Name(cluster=w129, "Start Time"=w127) -> (w128:T36)
        }
        frame "Reset All" {
        }
        frame "Config HW File Read" {
          n68 = Unbundle By Name(w136) -> ("Team Files Folder"=w133:path, "HW Config"=w135:T9)
          n69 = call "RWA_File Config.vim"("Read(f) Write(t)"=FALSE, "Target Folder Folder"=w133, "Any Config"=w135) -> ("Any Config Out"=w134:T9)  [unwired: 4 in, 4 out]
          n70 = Bundle By Name(cluster=w136, "HW Config"=w134, "Update Display"=TRUE) -> (w137:T36)
        }
        frame "Config HW File Save" {
          n71 = Unbundle By Name(w142) -> ("Team Files Folder"=w139:path, "HW Config"=w141:T9)
          n72 = call "RWA_File Config.vim"("Read(f) Write(t)"=TRUE, "Target Folder Folder"=w139, "Any Config"=w141) -> ("Any Config Out"=w140:T9)  [unwired: 4 in, 4 out]
          n73 = Bundle By Name(cluster=w142, "HW Config"=w140) -> (w143:T36)
        }
        frame "Config SW File Read" {
          n74 = Unbundle By Name(w149) -> ("Team Files Folder"=w146:path, "SW Config"=w148:T1)
          n75 = call "RWA_File Config.vim"("Read(f) Write(t)"=FALSE, "Target Folder Folder"=w146, "Any Config"=w148) -> ("Any Config Out"=w147:T1)  [unwired: 4 in, 4 out]
          n76 = Bundle By Name(cluster=w149, "SW Config"=w147, "Update Display"=TRUE) -> (w150:T36)
        }
        frame "Config SW File Save" {
          n77 = Unbundle By Name(w155) -> ("Team Files Folder"=w152:path, "SW Config"=w154:T1)
          n78 = call "RWA_File Config.vim"("Read(f) Write(t)"=TRUE, "Target Folder Folder"=w152, "Any Config"=w154) -> ("Any Config Out"=w153:T1)  [unwired: 4 in, 4 out]
          n79 = Bundle By Name(cluster=w155, "SW Config"=w153) -> (w156:T36)
        }
        frame "Config From FP" {
          n80 = Unbundle By Name(w163) -> ("HW Config"=w162:T9, "HW Config.WristHW Ver"=w159:u64)
          n81 = Unbundle By Name(w163) -> ("Current Time"=w172:timestamp)
          n82 = Unbundle By Name(w163) -> ("SW Config"=w165:T1, "SW Config.WristSW Ver"=w167:u64)
          n83 = call "Date Stamp.vi"("Time"=w172) -> ("U64 Out"=w158:u64)  [unwired: 5 in, 1 out]
          n84 = Not Equal?(x="HW Config", y=w162) -> (x != y?=w160:bool)
          n85 = Not Equal?(x=w165, y="SW Config") -> (x != y?=w168:bool)
          n86 = Select(t=w158, s=w168, f=w167) -> (s? t:f=w166:u64)
          n87 = Select(t=w158, s=w160, f=w159) -> (s? t:f=w157:u64)
          n88 = Bundle By Name(cluster="HW Config", "WristHW Ver"=w157) -> (w171:T9)
          n89 = Bundle By Name(cluster="SW Config", "WristSW Ver"=w166) -> (w170:T1)
          n90 = Bundle By Name(cluster=w163, "Update Display"=TRUE, "HW Config"=w171, "SW Config"=w170) -> (w173:T36)
        }
        frame "Config HW Get" {
          n91 = Unbundle By Name(w180) -> ("CANcoder Ref"=w175:T28, "Falcon Ref"=w184:T30, "HW Config"=w183:T9, "CAN Timeout"=w176:u32)
          n92 = Unbundle By Name(w183) -> ("CAN.Bus"=w182:string)
          n93 = call "Config HW Extract.vi"("Send Cmd Timout(ms)"=w176, "CANcoderRef"=w175, "CAN.Bus"=w182, "Wrist Config"=w183, "DevRef"=w184) -> ("Wrist Config Data Out"=w178:T9, "DevRef Out"=w179:T30, "CANcoderRef Out"=w174:T28)  [unwired: 3 in, 1 out]
          n94 = Bundle By Name(cluster=w180, "CANcoder Ref"=w174, "Falcon Ref"=w179, "HW Config"=w178, "Update Display"=TRUE) -> (w181:T36)
        }
        frame "Config HW Set" {
          n95 = Unbundle By Name(w191) -> ("CANcoder Ref"=w186:T28, "Falcon Ref"=w193:T30, "Max # Of Config Tries"=w187:i32, "HW Config"=w189:T9, "CAN Timeout"=w188:u32)
          n96 = call "Config HW Set.vi"("Send Cmd Timout(ms)"=w188, "CANcoder Ref"=w186, "Wrist Config"=w189, "Max # Of Tries"=w187, "DevRef"=w193) -> ("DevRef Out Out"=w190:T30, "CANcoder Ref Out"=w185:T28)  [unwired: 4 in, 1 out]
          n97 = Bundle By Name(cluster=w191, "CANcoder Ref"=w185, "Falcon Ref"=w190) -> (w192:T36)
        }
        frame "Open HW Only" {
          n98 = Unbundle By Name(w197) -> ("HW Config.CAN.Bus"=w196:string, "HW Config.CAN.ID"=w200:u8, "HW Config.Cancoder.ID"=w195:u8)
          n99 = call <vilib>:"CTRE_Phoenix_TalonFX_Open.vi"("Device Number"=w200, "CAN Bus"=w196) -> ("PhoenixMotorControlDevRef"=w199:T30)  [unwired: 8 in, 1 out]
          n100 = call <vilib>:"CTRE_Phoenix_CANcoder_Open.vi"("Device Number"=w195, "CAN Bus"=w196) -> ("CTRE_CANcoder_DeviceRef"=w194:T28)  [unwired: 8 in, 1 out]
          n101 = Bundle By Name(cluster=w197, "Falcon Ref"=w199, "CANcoder Ref"=w194) -> (w198:T36)
        }
        frame "Control FX Stop" {
          w202 = T29 0 items=["PercentOutput"=0, "Position"=1, "Velocity"=2, "Current"=3, "Follower"=5, "MotionProfile"=6, "MotionMagic"=7, "MotionProfileArc"=10, "Disabled"=15] ("FX Mode")
          n102 = Bundle By Name(cluster=w203, "FX Mode"=w202, "FX Set Value"=0.0) -> (w204:T36)
        }
        frame "Control FX Speed" {
          w207 = T29 0 items=["PercentOutput"=0, "Position"=1, "Velocity"=2, "Current"=3, "Follower"=5, "MotionProfile"=6, "MotionMagic"=7, "MotionProfileArc"=10, "Disabled"=15] ("FX Mode")
          n103 = Unbundle By Name(w206) -> ("ACT Input.Velocity (0-1)"=w205:dbl)
          n104 = Bundle By Name(cluster=w206, "FX Mode"=w207, "FX Set Value"=w205) -> (w208:T36)
        }
        frame "Control FX Positon" {
          w212 = T29 1 items=["PercentOutput"=0, "Position"=1, "Velocity"=2, "Current"=3, "Follower"=5, "MotionProfile"=6, "MotionMagic"=7, "MotionProfileArc"=10, "Disabled"=15] ("FX Mode")
          n105 = Unbundle By Name(w211) -> ("ACT Input.Position (counts)"=w209:i32)
          n106 = To Double Precision Float(number=w209) -> (double precision float=w210:dbl)
          n107 = Bundle By Name(cluster=w211, "FX Mode"=w212, "FX Set Value"=w210) -> (w213:T36)
        }
        frame "Config Cancoder Get Offset Value" {
          n108 = Unbundle By Name(w216) -> ("CANcoder Ref"=w218:T28)
          n109 = call-poly <vilib>:"CTRE_Phoenix_CANcoder_GetPolymorphic.vi"("CTRE_CANcoder_DeviceRef"=w218) -> ("Absolute Position"=w215:dbl)  [unwired: 10 in, 4 out]
          n110 = Bundle By Name(cluster=w216, "HW Config.Cancoder.Zero Offset"=w215, "Update Display"=TRUE) -> (w217:T36)
        }
      }
    }
    n111 = Unbundle By Name(w74) -> ("HW Config"=w71:T9, "Update Display"=w72:bool, "SW Config"=w42:T1)
    n112 = Unbundle By Name(w74) -> ("State"=w68:T35, "Falcon Ref"=w79:T30, "FX Mode"=w69:T29, "FX Set Value"=w70:dbl)
    n113 = Unbundle By Name(w74) -> ("Cycle Time(S)"=w76:dbl)
    "Cycle Time (S)" <- w76
    n114 = Unbundle By Name(w74) -> ("ACT Input"=→"CMD":T26, "HW Outputs"=w66:T3, "SW Outputs"=w51:T2)
    "HW Outputs" <- w66
    "SW Output" <- w51
    n115 = case shown="Default" w68 {
      tunnel: w79 -> [w116 w120]
      tunnel: [w116 w119] -> w78
      tunnel: w70 -> [_ w118]
      tunnel: w69 -> [_ w117]
      frame "Startup", "Configuring" {
      }
      frame Default {
        n116 = call <vilib>:"CTRE_Phoenix_MotorControl_Set.vi"("Output"=w118, "Control Mode"=w117, "PhoenixMotorControlDevRef"=w120) -> ("PhoenixMotorControlDevRef"=w119:T30)  [unwired: 7 in, 1 out]
      }
    }
    n117 = global write "Global_ACT_Data Out.vi" "ACT_Wrist_FX Mode"(w69) -> ()
    n118 = global write "Global_ACT_Data Out.vi" "ACT_Wrist_FX Value"(w70) -> ()
    n119 = case shown="False" w72 {
      tunnel: w71 -> [_ w122]
      tunnel: w42 -> [_ w121]
      frame False {
      }
      frame True {
        n120 = local write "SW Config"(w121) -> ()
        n121 = local write "HW Config"(w122) -> ()
      }
    }
    n122 = global write "Global_ACT_Data Out.vi" "ACT_Wrist_SW Output"(w51) -> ()
    n123 = global write "Global_ACT_Data Out.vi" "ACT_Wrist_HW Output"(w66) -> ()
    n124 = global write "Global_ACT_Data Out.vi" "ACT_Wrist_CycleTime(S)"(w76) -> ()
    n125 = Bundle By Name(cluster=w74, "Update Display"=FALSE, "Falcon Ref"=w78) -> (w77:T36)
  }
  n126 = flat-sequence {
    frame #0 {
      (unwired) ENUM_ACT_Action."Open HW Only" ("Action")
      (unwired) ENUM_ACT_State."Startup" ("State")
      (unwired) ENUM_ACT_Action."Config HW Get" ("Action")
      # "State LIST"
      # "Action LIST"
    }
  }
  n127 = Unbundle By Name(w19) -> ("Falcon Ref"=w7:T30)
  n128 = call <vilib>:"WPI_MotorControlClose.vi"("MotorControlDevRef"=w7) -> ()  [unwired: 10 in, 1 out]
